vi "16-RemoveLiteralPadding.vi"(11 "BITS in":bool[](array[boolean])) -> (3 "BITS out":bool[](array[boolean]))   [LabVIEW 2019, in "16.lvlib"]
uses:
  16.lvlib
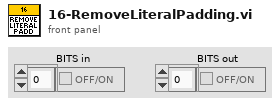
[diagram p1: front panel]
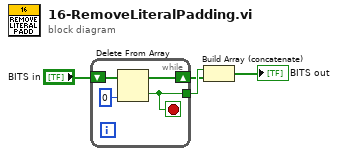
[diagram p0: block diagram]
diagram:
  n1 = while {
    shift-right: [w7] -> w2
    shift-left: "BITS in" -> [w8]
    tunnel: [w6] -> w4
    stop <- w6 stop-if-true
    n2 = Delete From Array(array=w8, index=0) -> (deleted portion=w6:bool, array with subset deleted=w7:bool[])  [unwired: 1 in]
  }
  n3 = Build Array (concatenate)(w4, w2) -> (→"BITS out":bool[])
